vi "paddleOcr_Openvino_easy.vi"() -> ()   [LabVIEW 2018]
uses:
  <vilib>/VIRobotics/opencv_yiku/ctls/RotatedRect.ctl
  <vilib>/VIRobotics/opencv_yiku/ctls/Point2f.ctl
  <vilib>/VIRobotics/opencv_yiku/ctls/Size2f.ctl
  <vilib>/VIRobotics/opencv_yiku/ctls/Size.ctl
  <vilib>/VIRobotics/opencv_yiku/ctls/ColorConversionCodes.ctl
  <vilib>/VIRobotics/ModelZoo/PaddleOCR/ppocr_openvino/ppocr_openvino.lvclass
  <vilib>/VIRobotics/opencv_yiku/Mat/Mat_8U/Mat_8U.lvclass
  <vilib>/VIRobotics/opencv_yiku/opencv_yiku.lvlib
panel:
  in  "backend":string="CPU"
  out "position":T1[](array[typedef])
  out "texts":string[](array[string])
  out "picture":picture
  in  "imgPath":path
  in  "PPOCRV5":string[](array[string])=["ppocrv5\\PP-OCRv5_server_det_infer.onnx", "ppocrv5\\PP-OCRv5_server_rec_infer.onnx", "cls\\cls.onnx", "ppocrv5\\ppocrv5_dict.txt"]
  in  "model_base_path":path=path "C:/ProgramData/VIRobotics/ModelZoo/PaddleOCR"
  # "Running PP-OCRv5 with OpenVINO in LabVIEW"
  # "You can replace “server” with “mobile”"
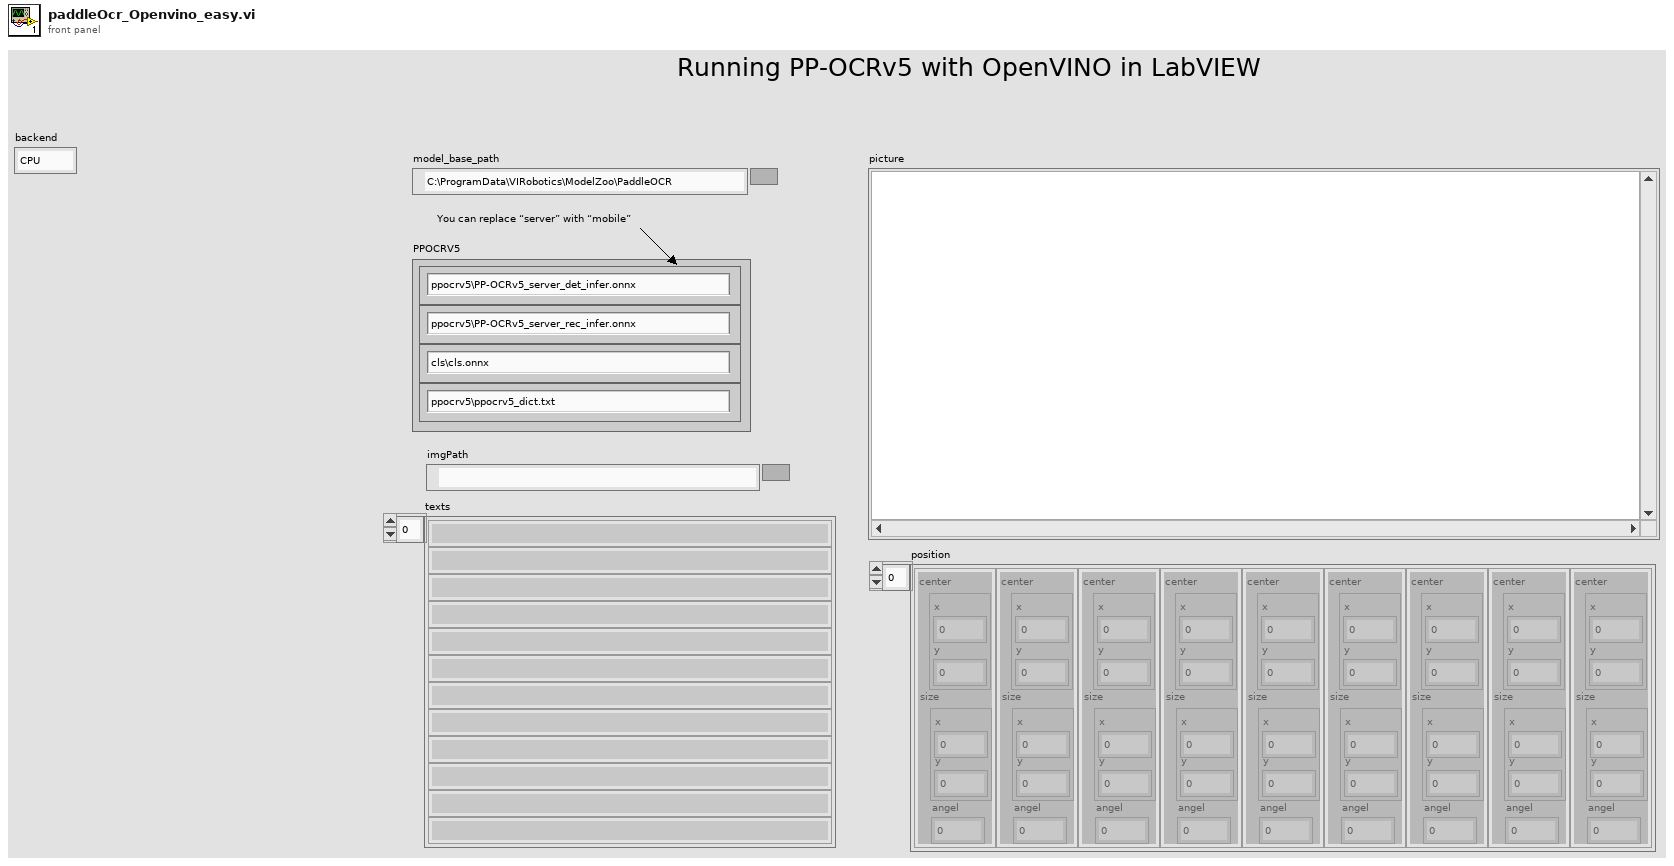
[diagram p1: front panel]
types:
  T1 = typedef "opencv_yiku.lvlib/RotatedRect.ctl" = cluster{"center":T2, "size":T3, "angel":sgl}
  T2 = typedef "opencv_yiku.lvlib/Point2f.ctl" = cluster{"x":sgl, "y":sgl}
  T3 = typedef "opencv_yiku.lvlib/Size2f.ctl" = cluster{"x":sgl, "y":sgl}
  T4 = cluster{"model_path":path, "backend":string, "deviceID":i32}
  T5 = typedef "opencv_yiku.lvlib/ColorConversionCodes.ctl" = enum32{"COLOR_BGR2BGRA", "COLOR_BGRA2BGR", "COLOR_BGR2RGBA", "COLOR_RGBA2BGR", "COLOR_BGR2RGB", "COLOR_BGRA2RGBA", "COLOR_BGR2GRAY", "COLOR_RGB2GRAY", "COLOR_GRAY2BGR", "COLOR_GRAY2BGRA", "COLOR_BGRA2GRAY", "COLOR_RGBA2GRAY", "COLOR_BGR2BGR565", "COLOR_RGB2BGR565", "COLOR_BGR5652BGR", "COLOR_BGR5652RGB", "COLOR_BGRA2BGR565", "COLOR_RGBA2BGR565", "COLOR_BGR5652BGRA", "COLOR_BGR5652RGBA", "COLOR_GRAY2BGR565", "COLOR_BGR5652GRAY", "COLOR_BGR2BGR555", "COLOR_RGB2BGR555", "COLOR_BGR5552BGR", "COLOR_BGR5552RGB", "COLOR_BGRA2BGR555", "COLOR_RGBA2BGR555", "COLOR_BGR5552BGRA", "COLOR_BGR5552RGBA", "COLOR_GRAY2BGR555", "COLOR_BGR5552GRAY", "COLOR_BGR2XYZ", "COLOR_RGB2XYZ", "COLOR_XYZ2BGR", "COLOR_XYZ2RGB", "COLOR_BGR2YCrCb", "COLOR_RGB2YCrCb", "COLOR_YCrCb2BGR", "COLOR_YCrCb2RGB", "COLOR_BGR2HSV", "COLOR_RGB2HSV", "42", "43", "COLOR_BGR2Lab", "COLOR_RGB2Lab"}
  T6 = typedef "opencv_yiku.lvlib/Size.ctl" = cluster{"x":i32, "y":i32}
  T7 = cluster{"[0]":cluster{"model_path":path, "backend":string, "deviceID":i32}, "[1]":cluster{"model_path":path, "backend":string, "deviceID":i32}, "[2]":cluster{"model_path":path, "backend":string, "deviceID":i32}, "[3]":cluster{"model_path":path, "backend":string, "deviceID":i32}}
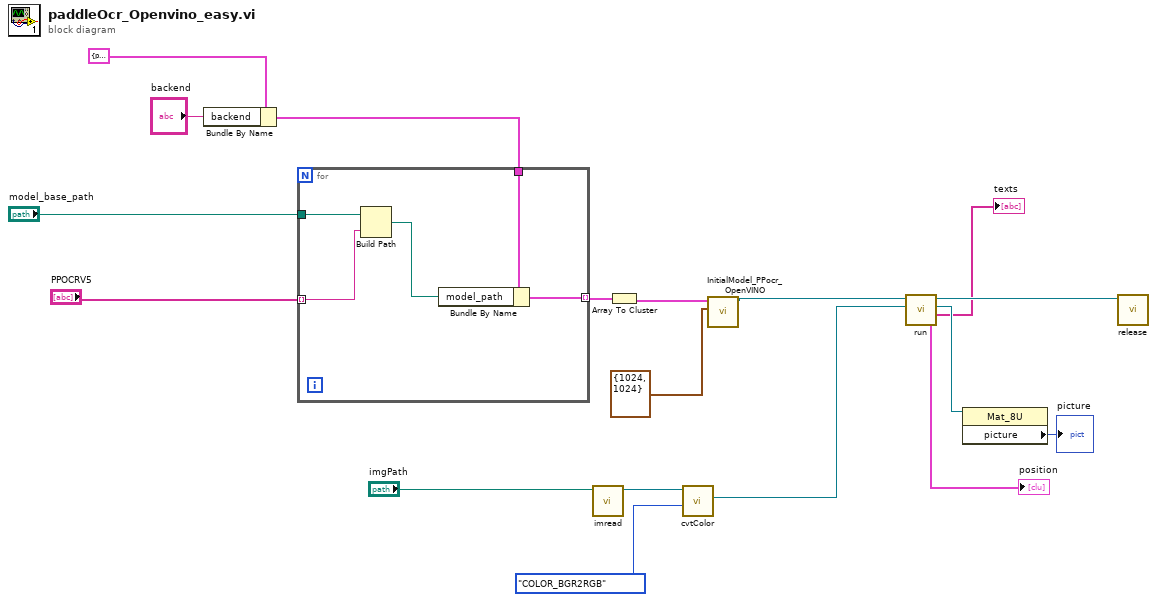
[diagram p0: block diagram]
diagram:
  n1 = Bundle By Name(cluster=T4 {"model_path"=path "", "backend"="CPU", "deviceID"=0} ("det"), "backend"="backend") -> (w3:T4)
  n2 = for {
    tunnel: w3 -> [w23]
    tunnel: "model_base_path" -> [w22]
    tunnel: "PPOCRV5" -> [w21] mode=indexing
    tunnel: [w19] -> w17 mode=indexing
    n3 = Build Path(base path=w22, name or relative path=w21) -> (appended path=w20:path)
    n4 = Bundle By Name(cluster=w23, "model_path"=w20) -> (w19:T4)
  }
  n5 = call <vilib>:"imread.vi"("path"="imgPath") -> ("Mat out"=w13:refnum<class "Mat_8U.lvclass">)  [unwired: 9 in, 1 out]
  n6 = Array To Cluster(array=w17) -> (cluster=w1:T7)
  n7 = call <vilib>:"cvtColor.vi"("dstCn"=ColorConversionCodes."COLOR_BGR2RGB", "src"=w13) -> ("dst out"=w11:refnum<class "Mat_8U.lvclass">)  [unwired: 7 in, 2 out]
  n8 = call <vilib>:"InitialModel_PPocr_OpenVINO.vi"("Size"=T6 {"x"=1024, "y"=1024}, "model_info"=w1) -> ("ppocr_onnx out"=w6:refnum<class "ppocr_openvino.lvclass">)  [unwired: 8 in, 1 out]
  n9 = call-dynamic "run.vi"("image"=w11, "OCR_Utils in"=w6) -> ("texts"=→"texts":string[], "image_out"=w10:refnum<class "Mat_8U.lvclass">, "OCR_Utils out"=w18:refnum<class "ppocr_openvino.lvclass">, "position"=→"position":T1[])  [unwired: 5 in, 1 out]
  n10 = property class="Mat_8U"(reference=w10) -> ("picture"=→"picture":picture)  [unwired: 1 in, 2 out]
  n11 = call-dynamic "release.vi"("OCR_Utils in"=w18) -> ()  [unwired: 9 in, 2 out]
